vi "Build Command Word.vi"(7 "Virtual Memory Unit in":refnum<class "Virtual Memory Unit.lvclass">, 8 "error in (no error)":errorcluster, 10 "Starting Address":u16 format="%04x", 11 "Message in":refnum<class "Message.lvclass">) -> (0 "error out":errorcluster, 2 "Next Available Address":u16 format="%04x", 3 "Message out":refnum<class "Message.lvclass">, 5 "Virtual Memory Unit out":refnum<class "Virtual Memory Unit.lvclass">)   [LabVIEW 2020, in "BCI-1553 API.lvlib" / "Message.lvclass"]
doc: "Sets up the message command word. This is the 1553 protocol word that will preface any data transactions required by this bus controller."
uses:
  Message.lvclass
  Dependencies/Virtual Memory Unit/Virtual Memory Unit.lvclass
  TypeDefs/Command Type.ctl
  Message.lvclass/Message.ctl
  BCI-1553 API.lvlib
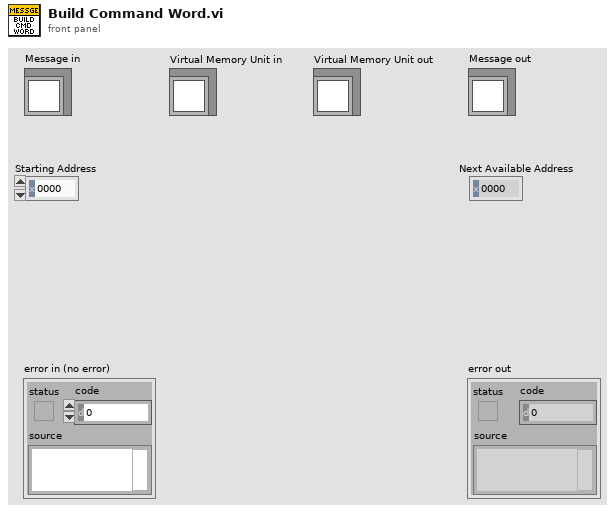
[diagram p1: front panel]
types:
  T1 = typedef "BCI-1553 API.lvlib/Command Type.ctl" = enum16{"Transmit", "Receive"}
  T2 = typedef "BCI-1553 API.lvlib/Command SubAddress.ctl" = enum16{"Mode Code", "1", "2", "3", "4", "5", "6", "7", "8", "9", "10", "11", "12", "13", "14", "15", "16", "17", "18", "19", "20", "21", "22", "23", "24", "25", "26", "27", "28", "29", "30"}
  T3 = typedef "BCI-1553 API.lvlib/Command Word Count.ctl" = enum16{"1", "2", "3", "4", "5", "6", "7", "8", "9", "10", "11", "12", "13", "14", "15", "16", "17", "18", "19", "20", "21", "22", "23", "24", "25", "26", "27", "28", "29", "30", "31", "32"}
  T4 = typedef "BCI-1553 API.lvlib/Command Terminal Address.ctl" = enum16{"0", "1", "2", "3", "4", "5", "6", "7", "8", "9", "10", "11", "12", "13", "14", "15", "16", "17", "18", "19", "20", "21", "22", "23", "24", "25", "26", "27", "28", "29", "30", "Broadcast"}
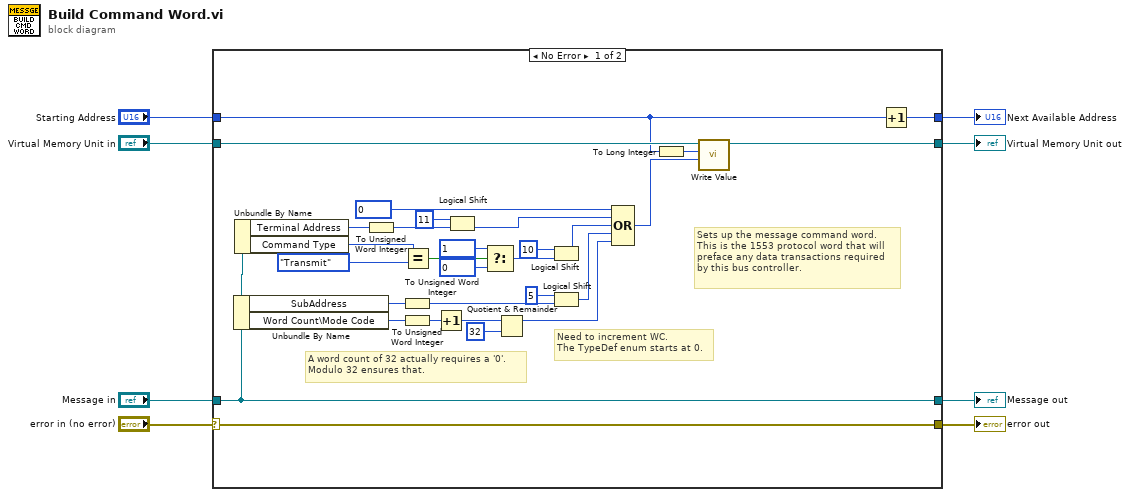
[diagram p0: block diagram]
diagram:
  n1 = case shown="No Error" "error in (no error)" {
    selector: "error in (no error)" -> [w38 w42]
    tunnel: [w38 w42] -> w7
    tunnel: [w31 w41] -> w5
    tunnel: "Message in" -> [w31 w41]
    tunnel: "Starting Address" -> [w15 w40]
    tunnel: "Virtual Memory Unit in" -> [w18 w39]
    tunnel: [w17 w39] -> w2
    tunnel: [w37 w40] -> w1
    frame No Error {
      # "Need to increment WC.\nThe TypeDef enum starts at 0."
      # "Sets up the message command word.\nThis is the 1553 protocol word that will\npreface any data transactions required\nby this bus controller."
      # "A word count of 32 actually requires a '0'.\nModulo 32 ensures that."
      n2 = Unbundle By Name(w31) -> ("SubAddress"=w23:T2, "Word Count\\Mode Code"=w19:T3)
      n3 = Unbundle By Name(w31) -> ("Terminal Address"=w35:T4, "Command Type"=w30:T1)
      n4 = To Unsigned Word Integer(number=w35) -> (unsigned 16bit integer=w13:u16)
      n5 = To Unsigned Word Integer(number=w23) -> (unsigned 16bit integer=w9:u16)
      n6 = To Unsigned Word Integer(number=w19) -> (unsigned 16bit integer=w12:u16)
      n7 = Equal?(x=w30, y=Command_Type."Transmit") -> (x = y?=w29:bool)
      n8 = Increment(x=w12) -> (x+1=w10:u16)
      n9 = Logical Shift(y=u16 11, x=w13) -> (x << y=w34:u16)
      n10 = Select(t=u16 1, s=w29, f=u16 0) -> (s? t:f=w26:u16)
      n11 = Quotient & Remainder(x=w10, y=u16 32) -> (x-y*floor(x/y)=w21:u16)  [unwired: 1 out]
      n12 = Logical Shift(y=i16 10, x=w26) -> (x << y=w25:u16)
      n13 = Logical Shift(y=u16 5, x=w9) -> (x << y=w22:u16)
      n14 = Compound Arithmetic op=OR(u16 0, w34, w25, w22, w21) -> (w16:u16)
      n15 = To Long Integer(number=w15) -> (32bit integer=w14:i32)
      n16 = call "Write Value.vi"("Value"=w16, "Index"=w14, "Virtual Memory Unit in"=w18) -> ("Virtual Memory Unit out"=w17:refnum<class "Virtual Memory Unit.lvclass">)  [unwired: 7 in, 1 out]
      n17 = Increment(x=w15) -> (x+1=w37:u16)
    }
    frame Error {
    }
  }
  "error out" <- w7
  "Message out" <- w5
  "Virtual Memory Unit out" <- w2
  "Next Available Address" <- w1
